vi "ChangeWavelengthGUI.vi"(4 "error in (no error)":errorcluster, 6 "Grating File":path) -> (0 "error out":errorcluster, 2 "Canceled?":bool, 3 "Wavelength Parameters Out":T3 {"Move type" items=["Both", "Grating Only", "Camera Only"]})   [LabVIEW 2015]
uses:
  wavelength_parameters.ctl
  movetypes.ctl
  GUI/GSP_GUI_global.vi
  GSP_Wavelength_Global.vi
panel:
  in  "Move type":T1 items=["Both", "Grating Only", "Camera Only"]
  in  "Camera Angle":dbl step=4.0
  in  "Change":bool
  in  "Grating Angle":dbl min=-0.01 max=45.0 step=2.0
  out "Grating Info":T2(array[cluster])
  in  "lines/mm":dbl
  out "Grating Info":string
  in  "Grating":i32(ring) items=["<NONE>", "RALC_1200", "<EMPTY>", "KOSI_600"]
  in  "Central Wavelength (nm)":dbl(knob) scale=350.0..900.0
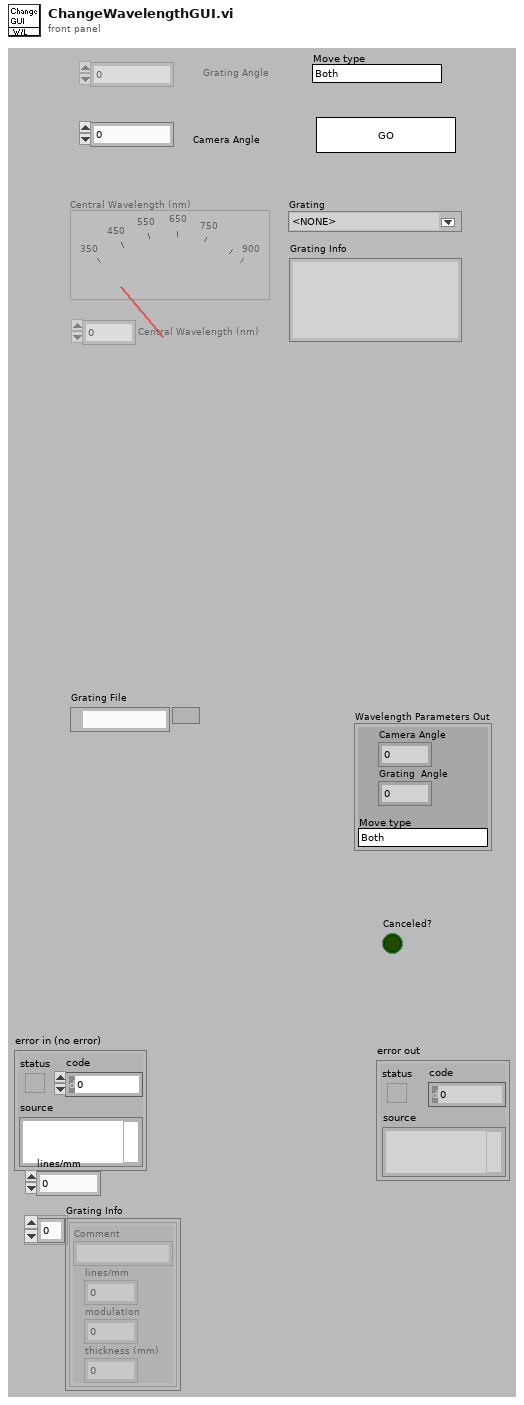
[diagram p1: front panel]
types:
  T1 = typedef "movetypes.ctl" = u16
  T2 = cluster{"Comment":string, "lines/mm":i32, "modulation":dbl, "thickness (mm)":dbl}[]
  T3 = typedef "wavelength_parameters.ctl" = cluster{"Camera Angle":dbl, "Grating  Angle":dbl, "Move type":T1}
  T4 = cluster{"Grating#":i32, "Slit#":i32, "Primary Filter#":i32, "Secondary Filter#":i32, "Coll Position":i32, "Camera Focus":i32, "Camera Angle":dbl, "Grating Angle":dbl, "Coll Temp":dbl, "CF Temp\n":dbl, "Camera Target":dbl, "Grating Target":dbl, "WAVMODE":string}
  T5 = cluster{"Comment":string, "lines/mm":i32, "modulation":dbl, "thickness (mm)":dbl}
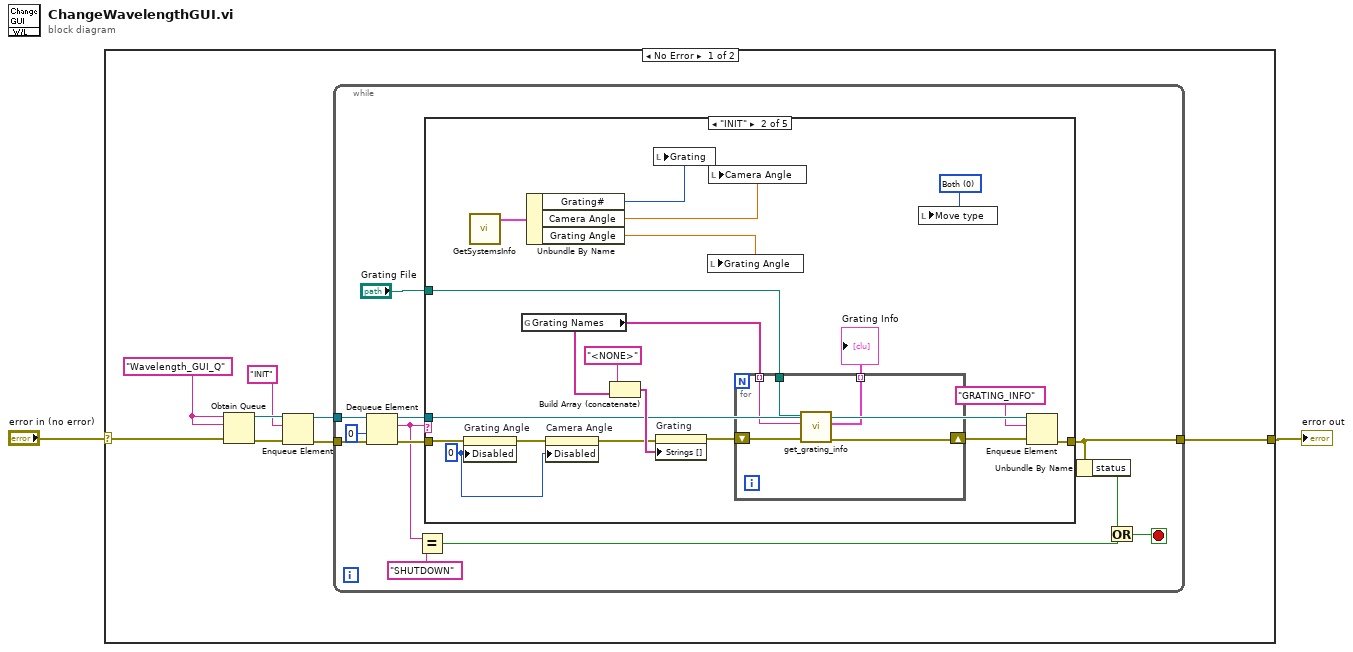
[diagram p0: block diagram]
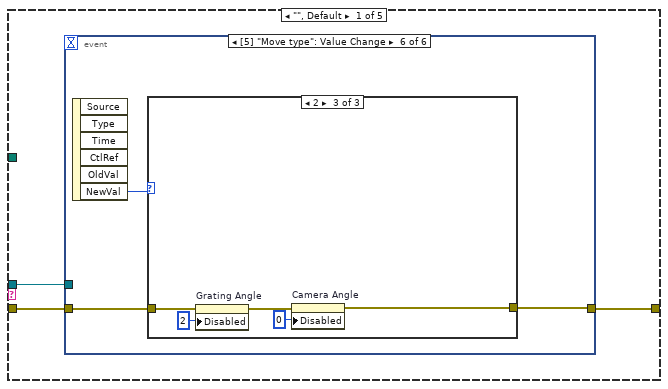
[diagram p2: hidden frame]
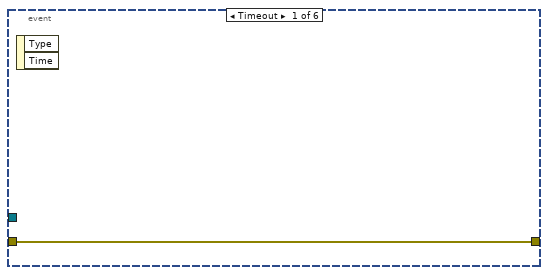
[diagram p3: hidden frame]
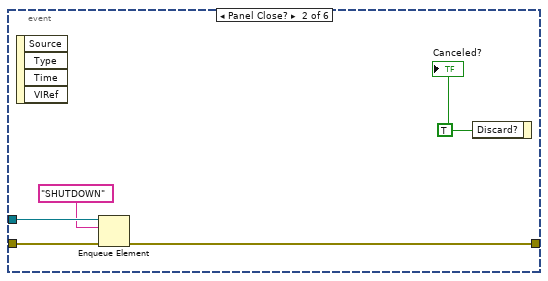
[diagram p4: hidden frame]
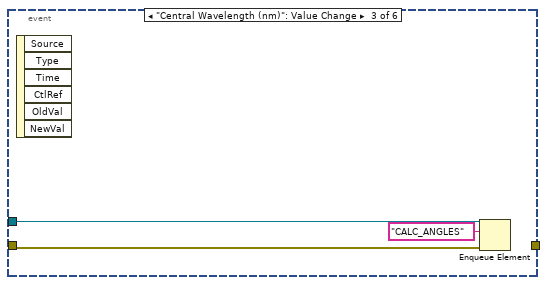
[diagram p5: hidden frame]
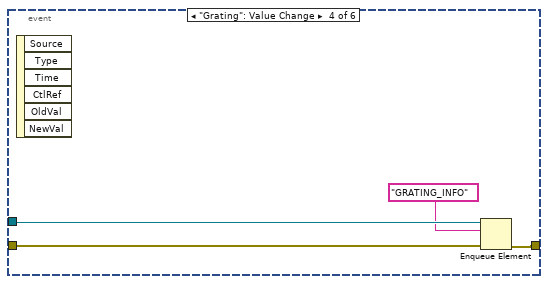
[diagram p6: hidden frame]
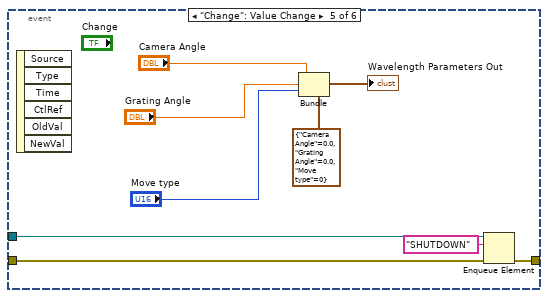
[diagram p7: hidden frame]
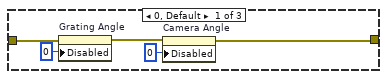
[diagram p8: hidden frame]
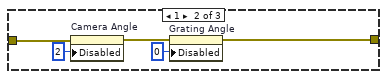
[diagram p9: hidden frame]
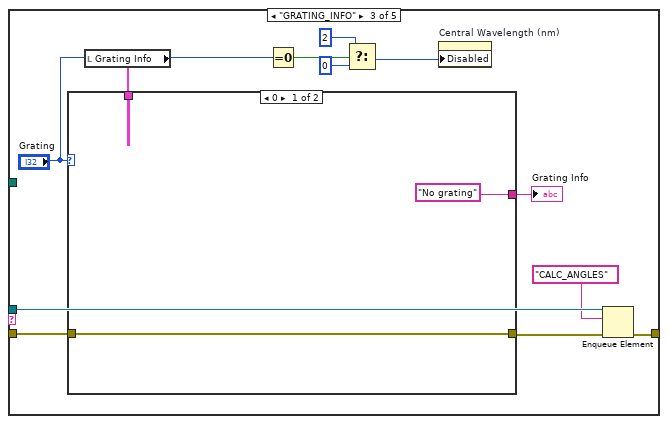
[diagram p10: hidden frame]
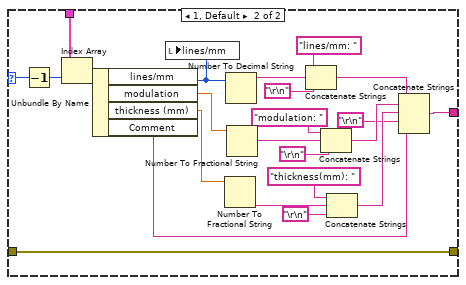
[diagram p11: hidden frame]
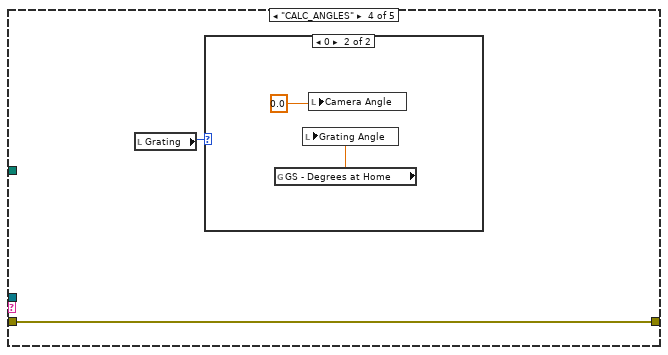
[diagram p12: hidden frame]
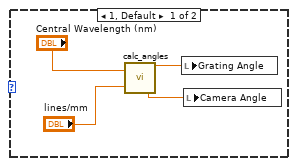
[diagram p13: hidden frame]
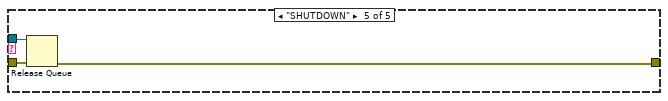
[diagram p14: hidden frame]
diagram:
  n1 = case shown="No Error" "error in (no error)" {
    selector: "error in (no error)" -> [w10 w138]
    tunnel: [w3 w138] -> w1
    frame No Error {
      w9 = "Wavelength_GUI_Q" ("name (unnamed)")
      n2 = Obtain Queue(name (unnamed)=w9, element data type=w9, error in (no error)=w10) -> (queue out=w8:refnum<queue>, error out=w7:errorcluster)  [unwired: 2 in, 1 out]
      n3 = Enqueue Element(queue=w8, element="INIT", error in (no error)=w7) -> (queue out=w5:refnum<queue>, error out=w4:errorcluster)  [unwired: 1 in, 1 out]
      n4 = while {
        tunnel: w5 -> [w22]
        tunnel: w4 -> [w21]
        tunnel: [w16] -> w3
        stop <- w14 stop-if-true
        n5 = Dequeue Element(queue=w22, timeout in ms (-1)=0, error in (no error)=w21) -> (queue out=w19:refnum<queue>, element=w18:string, error out=w20:errorcluster)  [unwired: 1 out]
        n6 = Equal?(x=w18, y="SHUTDOWN") -> (x = y?=w13:bool)
        n7 = case shown="\"INIT\"" w18 {
          tunnel: w20 -> [w24 w69 w101 w127 w136]
          tunnel: w19 -> [w25 w79 w96 _ w137]
          tunnel: [w23 w80 w98 w127 w135] -> w16
          tunnel: "Grating File" -> [_ w73 _ _ _]
          frame "", Default {
            n8 = event shown="[5] \"Move type\": Value Change" {
              selector: _ -> [_ _ _ _ _ _]
              dyn-events: _ -> [_ _ _ _ _ _]
              timeout: _ -> [_ _ _ _ _ _]
              tunnel: w25 -> [_ w30 w33 w37 w41 _]
              tunnel: w24 -> [w26 w29 w34 w36 w42 w50]
              tunnel: [w26 w27 _ w38 w43 w48] -> w23
              event Timeout {
                n9 = event-data() -> ()  [unwired: 1 in, 2 out]
              }
              event Panel Close? {
                w31 = TRUE
                n10 = event-data() -> ()  [unwired: 1 in, 4 out]
                n11 = Enqueue Element(queue=w30, element="SHUTDOWN", error in (no error)=w29) -> (error out=w27:errorcluster)  [unwired: 1 in, 2 out]
                n12 = event-data("Discard?"=w31) -> ()  [unwired: 1 in, 1 out]
                "Canceled?" <- w31
              }
              event "Central Wavelength (nm)": Value Change {
                n13 = event-data() -> ()  [unwired: 1 in, 6 out]
                n14 = Enqueue Element(queue=w33, element="CALC_ANGLES", error in (no error)=w34) -> ()  [unwired: 1 in, 3 out]
              }
              event "Grating": Value Change {
                n15 = event-data() -> ()  [unwired: 1 in, 6 out]
                n16 = Enqueue Element(queue=w37, element="GRATING_INFO", error in (no error)=w36) -> (error out=w38:errorcluster)  [unwired: 1 in, 2 out]
              }
              event "Change": Value Change {
                n17 = event-data() -> ()  [unwired: 1 in, 6 out]
                n18 = Bundle(cluster=T3 {"Camera Angle"=0.0, "Grating  Angle"=0.0, "Move type"=0} ("Wavelength Parameters Out"), "Camera Angle"="Camera Angle", "Grating  Angle"="Grating Angle", "Move type"="Move type") -> (→"Wavelength Parameters Out":T3)
                n19 = Enqueue Element(queue=w41, element="SHUTDOWN", error in (no error)=w42) -> (error out=w43:errorcluster)  [unwired: 1 in, 2 out]
              }
              event Value Change {
                n20 = event-data() -> ("NewVal"=w49:T1)  [unwired: 1 in, 5 out]
                n21 = case shown="2" w49 {
                  tunnel: w50 -> [w55 w60 w65]
                  tunnel: [w53 w56 w63] -> w48
                  frame 0, Default {
                    n22 = property on="Grating Angle" class="DigNum (strict)"(error in=w55, "Disabled"=u8 0) -> (error out=w54:errorcluster)  [unwired: 1 in, 1 out]
                    n23 = property on="Camera Angle" class="DigNum (strict)"(error in=w54, "Disabled"=u8 0) -> (error out=w53:errorcluster)  [unwired: 1 in, 1 out]
                  }
                  frame 1 {
                    n24 = property on="Camera Angle" class="DigNum (strict)"(error in=w60, "Disabled"=u8 2) -> (error out=w59:errorcluster)  [unwired: 1 in, 1 out]
                    n25 = property on="Grating Angle" class="DigNum (strict)"(error in=w59, "Disabled"=u8 0) -> (error out=w56:errorcluster)  [unwired: 1 in, 1 out]
                  }
                  frame 2 {
                    n26 = property on="Grating Angle" class="DigNum (strict)"(error in=w65, "Disabled"=u8 2) -> (error out=w64:errorcluster)  [unwired: 1 in, 1 out]
                    n27 = property on="Camera Angle" class="DigNum (strict)"(error in=w64, "Disabled"=u8 0) -> (error out=w63:errorcluster)  [unwired: 1 in, 1 out]
                  }
                }
              }
            }
          }
          frame "INIT" {
            w66 = u8 0 ("Disabled")
            w70 = T1 0 items=["Both", "Grating Only", "Camera Only"] ("Move type")
            n28 = property on="Grating Angle" class="DigNum (strict)"(error in=w69, "Disabled"=w66) -> (error out=w68:errorcluster)  [unwired: 1 in, 1 out]
            n29 = call "GetSystemsInfo.vi"() -> ("Pos Info"=w71:T4)
            n30 = global read "GSP_GUI_global.vi" "Grating Names"() -> (w74:string[])
            n31 = Unbundle By Name(w71) -> ("Grating#"=w72:i32, "Camera Angle"=w82:dbl, "Grating Angle"=w81:dbl)
            n32 = property on="Camera Angle" class="DigNum (strict)"(error in=w68, "Disabled"=w66) -> (error out=w67:errorcluster)  [unwired: 1 in, 1 out]
            n33 = Build Array (concatenate)("<NONE>" ("String"), w74) -> (w84:string[])
            n34 = local write "Grating"(w72) -> ()
            n35 = property on="Grating" class="Ring (strict)"(error in=w67, "Strings []"=w84) -> (error out=w77:errorcluster)  [unwired: 1 in, 1 out]
            n36 = local write "Grating Angle"(w81) -> ()
            n37 = local write "Camera Angle"(w82) -> ()
            n38 = for {
              tunnel: w73 -> [w89]
              shift-right: [w86] -> w76
              shift-left: w77 -> [w88]
              tunnel: [w87] -> w75 mode=indexing
              tunnel: w74 -> [w85] mode=indexing
              n39 = call "get_grating_info.vi"("error in (no error)"=w88, "grating name"=w85, "configuration file path"=w89) -> ("error out"=w86:errorcluster, "Grating Info"=w87:T5)  [unwired: 3 in]
            }
            "Grating Info" <- w75
            n40 = local write "Move type"(w70) -> ()
            n41 = Enqueue Element(queue=w79, element="GRATING_INFO", error in (no error)=w76) -> (error out=w80:errorcluster)  [unwired: 1 in, 2 out]
          }
          frame "GRATING_INFO" {
            n42 = local read "Grating Info"() -> (w100:T2)
            n43 = case shown="0" "Grating" {
              selector: "Grating" -> [_ w105]
              tunnel: w101 -> [w102 w106]
              tunnel: w100 -> [_ w126]
              tunnel: ["No grating" w108] -> w99
              tunnel: [w102 w106] -> w97
              frame 0 {
              }
              frame 1, Default {
                n44 = Decrement(x=w105) -> (x-1=w104:i32)
                n45 = Index Array(array=w126, index=w104) -> (element=w125:T5)
                n46 = Unbundle By Name(w125) -> ("lines/mm"=w107:i32, "modulation"=w111:dbl, "thickness (mm)"=w110:dbl, "Comment"=w109:string)
                n47 = local write "lines/mm"(w107) -> ()
                n48 = Number To Fractional String(number=w110) -> (F-format string=w112:string)  [unwired: 3 in]
                n49 = Number To Decimal String(number=w107) -> (decimal integer string=w124:string)  [unwired: 1 in]
                n50 = Number To Fractional String(number=w111) -> (F-format string=w120:string)  [unwired: 3 in]
                n51 = Concatenate Strings("lines/mm: ", w124, "\r\n") -> (w116:string)
                n52 = Concatenate Strings("modulation: " ("string"), w120, "\r\n") -> (w115:string)
                n53 = Concatenate Strings("thickness(mm): " ("string"), w112, "\r\n") -> (w114:string)
                n54 = Concatenate Strings(w116, w115, w114, "\r\n", w109) -> (w108:string)
              }
            }
            "Grating Info" <- w99
            n55 = Equal To 0?(x="Grating") -> (x = 0?=w93:bool)
            n56 = Select(t=u8 2 ("Disabled"), s=w93, f=u8 0) -> (s? t:f=w90:u8)
            n57 = property on="Central Wavelength (nm)" class="Knob (strict)"("Disabled"=w90) -> ()  [unwired: 2 in, 2 out]
            n58 = Enqueue Element(queue=w96, element="CALC_ANGLES", error in (no error)=w97) -> (error out=w98:errorcluster)  [unwired: 1 in, 2 out]
          }
          frame "CALC_ANGLES" {
            n59 = local read "Grating"() -> (w128:i32)
            n60 = case shown="0" w128 {
              frame 1, Default {
                n61 = call "calc_angles.vi"("lines/mm"="lines/mm", "Central Wavlength (nm)"="Central Wavelength (nm)") -> ("camera angle"=w130:dbl, "grating angle"=w131:dbl)
                n62 = local write "Grating Angle"(w131) -> ()
                n63 = local write "Camera Angle"(w130) -> ()
              }
              frame 0 {
                n64 = global read "GSP_Wavelength_Global.vi" "GS - Degrees at Home"() -> (w133:dbl)
                n65 = local write "Grating Angle"(w133) -> ()
                n66 = local write "Camera Angle"(0.0) -> ()
              }
            }
          }
          frame "SHUTDOWN" {
            n67 = Release Queue(queue=w137, error in (no error)=w136) -> (error out=w135:errorcluster)  [unwired: 1 in, 2 out]
          }
        }
        n68 = Unbundle By Name(w16) -> ("status"=w15:bool)
        n69 = Or(x=w15, y=w13) -> (x .or. y?=w14:bool)
      }
    }
    frame Error {
    }
  }
  "error out" <- w1
